vi "Step ADD ACW W Parameters.vi"(0 "VISA resource name":refnum<visa-resource-name>, 1 "ACW Test Parameters":T2={"Voltage (1240)"=1240, "High Limit Total (10)"=5.0, "Low Limit Total (0)"=0.0, "High Limit Real(10)"=10.0, "Low Limit Real (0)"=0.0, "Ramp Up Time (0.1 - 999.9 seconds) (0.1)"=0.1, "Dwell Time (0, 0.2 - 999.9 seconds) (1)"=1.0, "Ramp Down Time (0.0 - 999.9 seconds) (1)"=0.0, "Arc Sense (1 - 9) (5)"=5, "Arc Detect (F: Off)"=FALSE, "Continuity (F: Off)"=FALSE, "Range  "=enum."AUTO", "Offset (0)"=0.0, "Auto Offset (F: Off)"=FALSE, "Frequency"=enum."60"} {"Offset (0)" format="%.2f"; "Ramp Down Time (0.0 - 999.9 seconds) (1)" format="%.1f"; "Low Limit Real (0)" format="%.3f"; "High Limit Real(10)" format="%.2f"; "Dwell Time (0, 0.2 - 999.9 seconds) (1)" format="%.1f"; "Ramp Up Time (0.1 - 999.9 seconds) (0.1)" format="%.1f"; "Low Limit Total (0)" format="%.3f"; "High Limit Total (10)" format="%.2f"; "Voltage (1240)" min=0 max=12000}, 2 "Internal scanner?":bool, 3 "Scanner Settings":T1={"Scan1"=1, "Scan2"=1, "Scan3"=1, "Scan4"=1, "Scan5"=1, "Scan6"=1, "Scan7"=1, "Scan8"=1, "Scan9"=1, "Scan10"=1, "Scan11"=1, "Scan12"=1, "Scan13"=1, "Scan14"=1, "Scan15"=1, "Scan16"=1} {"Scan16" scale=0.0..2.0; "Scan15" scale=0.0..2.0; "Scan14" scale=0.0..2.0; "Scan13" scale=0.0..2.0; "Scan12" scale=0.0..2.0; "Scan11" scale=0.0..2.0; "Scan10" scale=0.0..2.0; "Scan9" scale=0.0..2.0; "Scan8" scale=0.0..2.0; "Scan7" scale=0.0..2.0; "Scan6" scale=0.0..2.0; "Scan5" scale=0.0..2.0; "Scan4" scale=0.0..2.0; "Scan3" min=0 max=2 scale=0.0..2.0; "Scan2" min=0 max=2 scale=0.0..2.0; "Scan1" min=0 max=2 scale=0.0..2.0}, 7 "Step Selection (1-200)":i32=1, 9 "Add Step":bool, 11 "error in (no error)":errorcluster) -> (4 "VISA resource name out":refnum<visa-resource-name>, 15 "error out":errorcluster)   [LabVIEW 2020, in "Associated Research 78XX Series.lvlib"]
doc: "Set the desired memory location to ACW mode with the specified parameters."
uses:
  <instrlib>/Associated Research 78XX Series/Associated Research 78XX Series.lvlib
  <instrlib>/Associated Research 78XX Series/Public/Configure/Steps/Low Level/ACW Test Parameters.ctl
  <instrlib>/Associated Research 78XX Series/Public/Configure/Steps/Low Level/Scanner Settings.ctl
panel:
  # "Add"
  # "Edit"
  # "On\nOff"
  # "On\nOff"
  # "On\nOff"
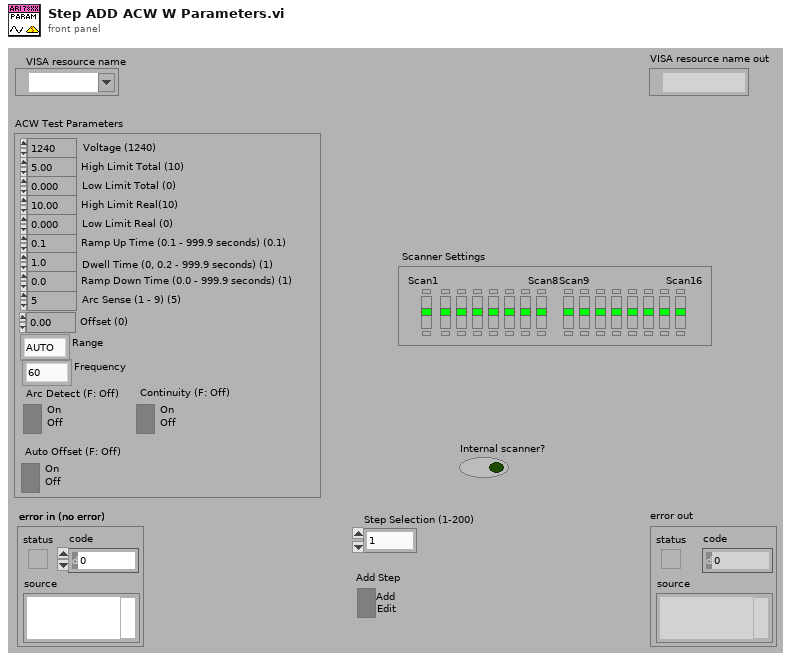
[diagram p1: front panel]
types:
  T1 = typedef "Associated Research 78XX Series.lvlib/Scanner Settings.ctl" = cluster{"Scan1":i32, "Scan2":i32, "Scan3":i32, "Scan4":i32, "Scan5":i32, "Scan6":i32, "Scan7":i32, "Scan8":i32, "Scan9":i32, "Scan10":i32, "Scan11":i32, "Scan12":i32, "Scan13":i32, "Scan14":i32, "Scan15":i32, "Scan16":i32}
  T2 = typedef "Associated Research 78XX Series.lvlib/ACW Test Parameters.ctl" = cluster{"Voltage (1240)":i32, "High Limit Total (10)":dbl, "Low Limit Total (0)":dbl, "High Limit Real(10)":dbl, "Low Limit Real (0)":dbl, "Ramp Up Time (0.1 - 999.9 seconds) (0.1)":dbl, "Dwell Time (0, 0.2 - 999.9 seconds) (1)":dbl, "Ramp Down Time (0.0 - 999.9 seconds) (1)":dbl, "Arc Sense (1 - 9) (5)":i32, "Arc Detect (F: Off)":bool, "Continuity (F: Off)":bool, "Range  ":enum16{"AUTO", "FIXED"}, "Offset (0)":dbl, "Auto Offset (F: Off)":bool, "Frequency":enum16{"50", "60", "400", "800"}}
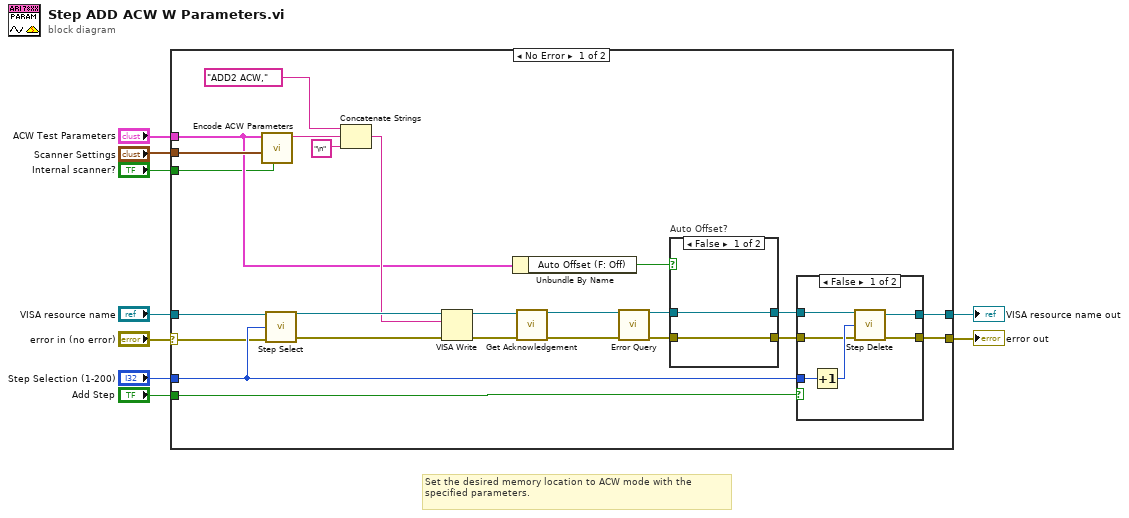
[diagram p0: block diagram]
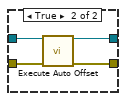
[diagram p2: hidden frame]
diagram:
  # "Set the desired memory location to ACW mode with the specified parameters."
  n1 = case shown="No Error" "error in (no error)" {
    selector: "error in (no error)" -> [w15 w49]
    tunnel: [w31 w49] -> w8
    tunnel: [w30 w48] -> w6
    tunnel: "VISA resource name" -> [w16 w48]
    tunnel: "Step Selection (1-200)" -> [w17 _]
    tunnel: "Add Step" -> [w29 _]
    tunnel: "ACW Test Parameters" -> [w18 _]
    tunnel: "Scanner Settings" -> [w19 _]
    tunnel: "Internal scanner?" -> [w13 _]
    frame No Error {
      n2 = call <instrlib>:"Encode ACW Parameters.vi"("scanner?"=w13, "Scanner Settings"=w19, "ACW Test Parameters in"=w18) -> ("ADD Parameters"=w10:string)  [unwired: 6 in, 2 out]
      n3 = call <instrlib>:"Step Select.vi"("VISA resource name"=w16, "Step Number (1)"=w17, "error in (no error)"=w15) -> ("VISA resource name out"=w32:refnum<visa-resource-name>, "error out"=w33:errorcluster)  [unwired: 11 in]
      n4 = Concatenate Strings("ADD2 ACW," ("string"), w10, "\n" ("string")) -> (w27:string)
      n5 = VISA Write(VISA resource name=w32, write buffer=w27, error in (no error)=w33) -> (VISA resource name out=w12:refnum<visa-resource-name>, error out=w11:errorcluster)  [unwired: 1 out]
      n6 = Unbundle By Name(w18) -> ("Auto Offset (F: Off)"=w24:bool)
      n7 = call <instrlib>:"Get Acknowledgement.vi"("VISA resource name"=w12, "error in (no error)"=w11) -> ("VISA resource name out"=w26:refnum<visa-resource-name>, "error out"=w25:errorcluster)  [unwired: 12 in]
      n8 = call <instrlib>:"Error Query.vi"("VISA resource name"=w26, "error in (no error)"=w25) -> ("VISA resource name out"=w23:refnum<visa-resource-name>, "error out"=w22:errorcluster)  [unwired: 10 in, 2 out]
      n9 = case "Auto Offset?" shown="False" w24 {
        tunnel: w23 -> [w35 w36]
        tunnel: w22 -> [w34 w37]
        tunnel: [w34 w38] -> w20
        tunnel: [w35 w39] -> w21
        frame False {
        }
        frame True {
          n10 = call <instrlib>:"Execute Auto Offset.vi"("VISA resource name"=w36, "error in (no error)"=w37) -> ("VISA resource name out"=w39:refnum<visa-resource-name>, "error out"=w38:errorcluster)  [unwired: 12 in]
        }
      }
      n11 = case shown="False" w29 {
        tunnel: w17 -> [w45 _]
        tunnel: w20 -> [w43 w46]
        tunnel: w21 -> [w42 w47]
        tunnel: [w41 w46] -> w31
        tunnel: [w40 w47] -> w30
        frame False {
          n12 = Increment(x=w45) -> (x+1=w44:i32)
          n13 = call <instrlib>:"Step Delete.vi"("VISA resource name"=w42, "Step Number (0 = Active Step)"=w44, "error in (no error)"=w43) -> ("VISA resource name out"=w40:refnum<visa-resource-name>, "error out"=w41:errorcluster)  [unwired: 11 in]
        }
        frame True {
        }
      }
    }
    frame Error {
    }
  }
  "error out" <- w8
  "VISA resource name out" <- w6
